vi "ep_Event Limits.vi"(8 "error in (no error)":errorcluster, 10 "reference voltages":dbl[](array[numeric]), 11 "events settings":T2={"swell threshold [%]"=110.0, "dip threshold [%]"=90.0, "interruption threshold [%]"=1.0, "hysteresis [%]"=2.0}) -> (0 "error out":errorcluster, 3 "event limits":T1(array[cluster]))   [LabVIEW 2014, in "NI_EP_Power Quality.lvlib"]
uses:
  <vilib>/addons/Electrical Power/PQ/NI_EP_Power Quality.lvlib
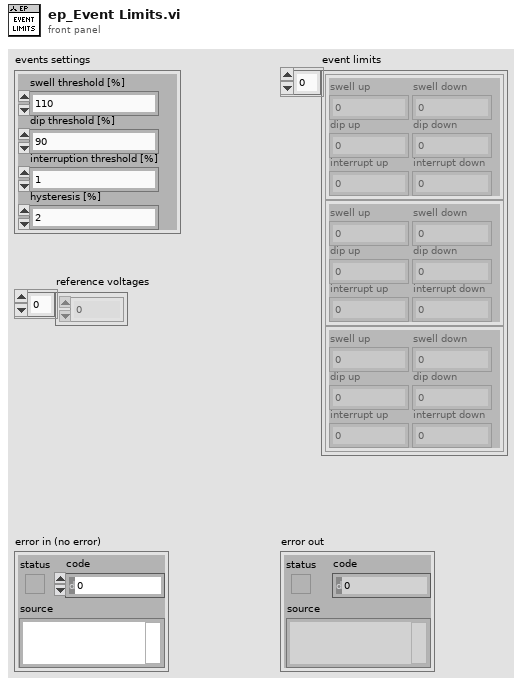
[diagram p1: front panel]
types:
  T1 = cluster{"swell up":dbl, "swell down":dbl, "dip up":dbl, "dip down":dbl, "interrupt up":dbl, "interrupt down":dbl}[]
  T2 = cluster{"swell threshold [%]":dbl, "dip threshold [%]":dbl, "interruption threshold [%]":dbl, "hysteresis [%]":dbl}
  T3 = cluster{"swell up":dbl, "swell down":dbl, "dip up":dbl, "dip down":dbl, "interrupt up":dbl, "interrupt down":dbl}
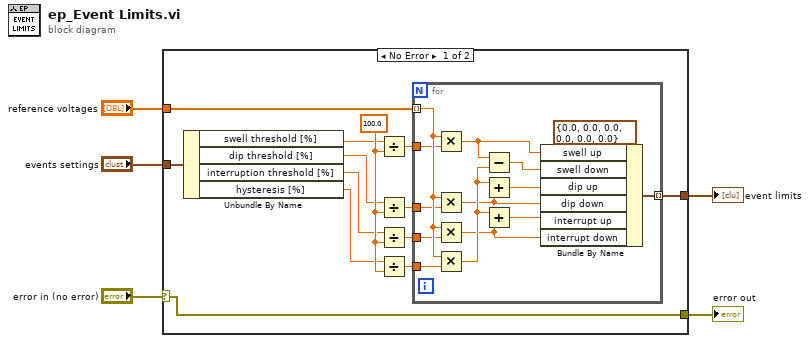
[diagram p0: block diagram]
diagram:
  n1 = case shown="No Error" "error in (no error)" {
    selector: "error in (no error)" -> [w6 w33]
    tunnel: "reference voltages" -> [w18 _]
    tunnel: "events settings" -> [w17 _]
    tunnel: [w16 _] -> w3
    tunnel: [w6 w33] -> w1
    frame No Error {
      w15 = 100.0
      n2 = Unbundle By Name(w17) -> ("swell threshold [%]"=w14:dbl, "dip threshold [%]"=w13:dbl, "interruption threshold [%]"=w12:dbl, "hysteresis [%]"=w11:dbl)
      n3 = Divide(x=w14, y=w15) -> (x/y=w10:dbl)
      n4 = Divide(x=w13, y=w15) -> (x/y=w9:dbl)
      n5 = Divide(x=w12, y=w15) -> (x/y=w8:dbl)
      n6 = Divide(x=w11, y=w15) -> (x/y=w7:dbl)
      n7 = for {
        tunnel: w18 -> [w31] mode=indexing
        tunnel: [w32] -> w16 mode=indexing
        tunnel: w10 -> [w28]
        tunnel: w9 -> [w27]
        tunnel: w8 -> [w26]
        tunnel: w7 -> [w25]
        n8 = Multiply(x=w31, y=w28) -> (x*y=w20:dbl)
        n9 = Multiply(x=w31, y=w27) -> (x*y=w22:dbl)
        n10 = Multiply(x=w31, y=w26) -> (x*y=w21:dbl)
        n11 = Multiply(x=w31, y=w25) -> (x*y=w23:dbl)
        n12 = Subtract(x=w20, y=w23) -> (x-y=w19:dbl)
        n13 = Add(x=w23, y=w22) -> (x+y=w30:dbl)
        n14 = Add(x=w23, y=w21) -> (x+y=w29:dbl)
        n15 = Bundle By Name(cluster=T3 {"swell up"=0.0, "swell down"=0.0, "dip up"=0.0, "dip down"=0.0, "interrupt up"=0.0, "interrupt down"=0.0} ("event limits"), "swell up"=w20, "swell down"=w19, "dip up"=w30, "dip down"=w22, "interrupt up"=w29, "interrupt down"=w21) -> (w32:T3)
      }
    }
    frame Error {
    }
  }
  "event limits" <- w3
  "error out" <- w1
